vi "Event handler-Z Setup.vi"(8 "error in (no error)":errorcluster, 9 "Obtain Z Stop":bool, 11 "Obtain Z Start":bool) -> (0 "error out":errorcluster)   [LabVIEW 2017]
uses:
  Typedefs/Read Write Enum.ctl
  Global Variables/gl_UI Ctrl Refs.vi
  Global Variables/General Globals.vi
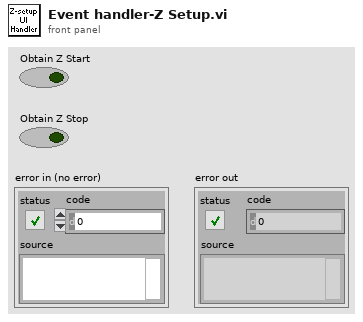
[diagram p1: front panel]
types:
  T1 = typedef "Read Write Enum.ctl" = enum16{"Read", "Write"}
  T2 = typedef "UI ctrl refs cluster.ctl" = cluster{"Top level VI path":path, "Top level VI ref":refnum<vi>, "User menu ref":refnum<k9>, "Sub Panel control":refnum<vi>, "Imaging Param Tab":refnum<vi>, "Occurrence-Start drivers":refnum<k4>, "Occurrence-Speed logging initialised":refnum<k4>, "Occurrence-XYZ stage initialised":refnum<k4>, "Exit button":refnum<vi>, "Status ind":refnum<vi>, "Set as origin":refnum<vi>, "Speed Logging":refnum<vi>, "Time Lapse":refnum<vi>, "Live Imaging":refnum<vi>, "AOL Z Stack":refnum<vi>, "Motor Z Stack":refnum<vi>, "Funct Acq button":refnum<vi>, "Hard Shutter":refnum<vi>, "Virtual Shutter":refnum<vi>, "Laser Power":refnum<vi>, "AOL Mode":refnum<vi>, "Frame Size":refnum<vi>, "Field of View":refnum<vi>, "Dwell Time":refnum<vi>, "Zoom":refnum<vi>, "AOL Z":refnum<vi>, "Objective":refnum<vi>, "Axis":refnum<vi>, "Paths & Names":refnum<vi>, "Experiment folder path (ind.)":refnum<vi>, "Last State (Ind.)":refnum<vi>, "Averages":refnum<vi>, "Angle (degrees)":refnum<vi>, "X centre":refnum<vi>, "Y centre":refnum<vi>, "Plane Mode":refnum<vi>, "# Planes":refnum<vi>, "Z Start":refnum<vi>, "Z Stop":refnum<vi>, "Z Step":refnum<vi>, "PMT 1":refnum<vi>, "PMT 2":refnum<vi>, "Stage XYZ Position":refnum<vi>, "Pockels@Z Start":refnum<vi>, "Pockels@Z Stop":refnum<vi>, "Obtain Z Start":refnum<vi>, "Obtain Z Stop":refnum<vi>, "Live stim.trig.period":refnum<vi>, "Live stim.trig.enable":refnum<vi>, "Movement Correction":refnum<vi>, "Load Reference Image":refnum<vi>, "XY Stage Move":refnum<vi>, "MovCor Cluster":refnum<vi>, "RefDAQParam":refnum<vi>, "Funct. Acq. Pockels Modulation":refnum<vi>, "Ref Laser Power":refnum<vi>, "Enable Video Recording":refnum<vi>, "Video Record-Live Imaging":refnum<vi>, "Video Record-Funct acq":refnum<vi>, "Reference Source":refnum<vi>, "AOL Z-stack Chirps Ready (ind)":refnum<vi>, "Target time between mov.cor. ref triggers (ms)":refnum<vi>, "Funct. Acq. Ref frame save":refnum<vi>, "Tracking button":refnum<vi>, "Show ref plots window":refnum<vi>, "Center freq ind (nm)":refnum<vi>, "Pickup mode (ind)":refnum<vi>, "Logging queue (ind)":refnum<vi>, "Back aperture power (ind.)":refnum<vi>, "Power after objective (ind.)":refnum<vi>, "Switch user":refnum<vi>, "Ls1 Conn. Status":refnum<vi>, "Ls1Tuning Status":refnum<vi>, "Ls1 Faults":refnum<vi>, "Ls1 Connection":refnum<vi>, "Ls1 Mode":refnum<vi>, "Ls1 POWER [mW]":refnum<vi>, "Ls1Shutter":refnum<vi>, "Ls1 Wavelength":refnum<vi>, "Ls1 Note":refnum<vi>, "Ls1 Confirm Wav":refnum<vi>, "Ls1 PreChrp Prism1":refnum<vi>, "Ls1 PreChrp Prism2":refnum<vi>, "Ls1 wav top Ind":refnum<vi>, "Ls1 power top Ind":refnum<vi>, "Ls1 Pump peak Hold":refnum<vi>, "Ls1 Status Ind":refnum<vi>, "Ls1 wav cancel":refnum<vi>, "Experiment Type":refnum<vi>, "Biology Information":refnum<vi>}
  T3 = typedef "Laser control knob.ctl" = u16
  T4 = cluster{"ZStack":cluster{"Zstart":dbl, "Zstop":dbl, "Zstep":dbl}, "Laser Power %":cluster{"@ Start":dbl, "@ Stop":dbl}}
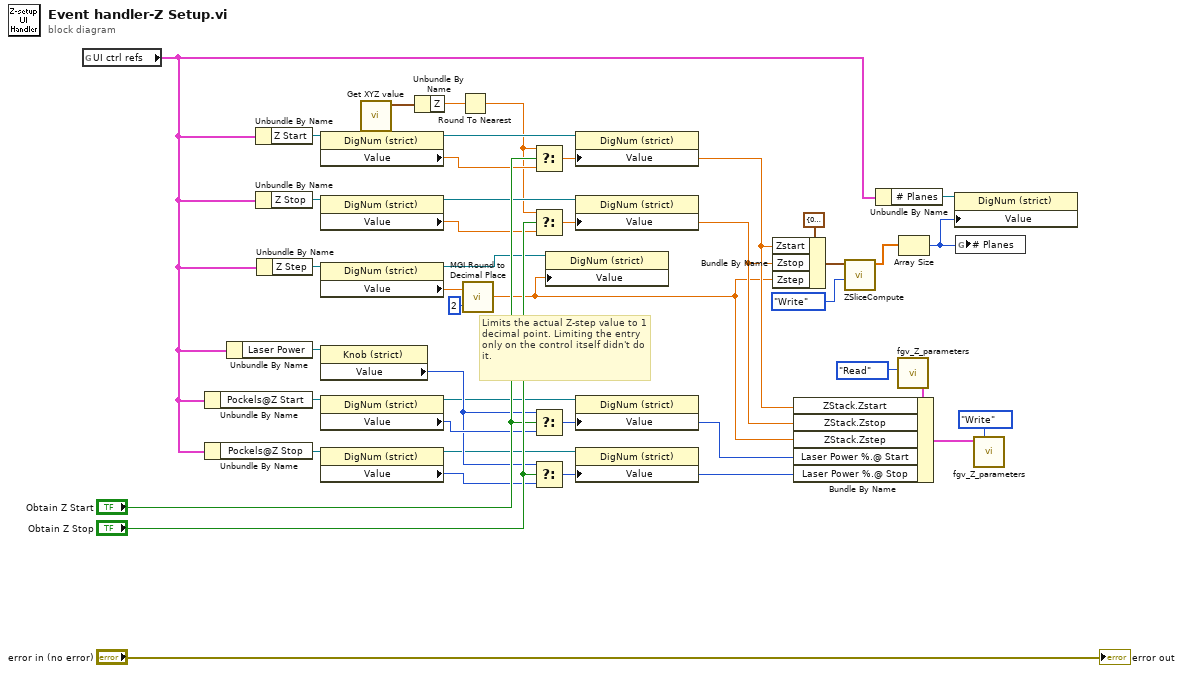
[diagram p0: block diagram]
diagram:
  # "Limits the actual Z-step value to 1 decimal point. Limiting the entry only on the control itself didn't do it."
  n1 = global read "gl_UI Ctrl Refs.vi" "UI ctrl refs"() -> (w38:T2)
  n2 = Unbundle By Name(w38) -> ("Pockels@Z Start"=w16:refnum<vi>)
  n3 = Unbundle By Name(w38) -> ("Pockels@Z Stop"=w15:refnum<vi>)
  n4 = Unbundle By Name(w38) -> ("Laser Power"=w17:refnum<vi>)
  n5 = Unbundle By Name(w38) -> ("Z Start"=w23:refnum<vi>)
  n6 = Unbundle By Name(w38) -> ("Z Stop"=w22:refnum<vi>)
  n7 = Unbundle By Name(w38) -> ("Z Step"=w18:refnum<vi>)
  n8 = property on="Property Node" class="DigNum (strict)"(reference=w23) -> (reference out=w26:refnum<vi>, "Value"=w25:dbl)  [unwired: 1 in, 1 out]
  n9 = property on="Property Node" class="DigNum (strict)"(reference=w22) -> (reference out=w21:refnum<vi>, "Value"=w20:dbl)  [unwired: 1 in, 1 out]
  n10 = property on="Property Node" class="DigNum (strict)"(reference=w18) -> (reference out=w2:refnum<vi>, "Value"=w3:dbl)  [unwired: 1 in, 1 out]
  n11 = property on="Property Node" class="Knob (strict)"(reference=w17) -> ("Value"=w32:T3)  [unwired: 1 in, 2 out]
  n12 = property on="Property Node" class="DigNum (strict)"(reference=w16) -> (reference out=w14:refnum<vi>, "Value"=w33:u16)  [unwired: 1 in, 1 out]
  n13 = property on="Property Node" class="DigNum (strict)"(reference=w15) -> (reference out=w13:refnum<vi>, "Value"=w31:u16)  [unwired: 1 in, 1 out]
  n14 = call "Get XYZ value.vi"() -> ("Stage XYZ Position"=w7:cluster{"X":sgl, "Y":sgl, "Z":sgl})  [unwired: 11 in]
  n15 = Unbundle By Name(w7) -> ("Z"=w34:sgl)
  n16 = Round To Nearest(number=w34) -> (nearest integer value=w5:sgl)
  n17 = call <userlib>:"MGI Round to Decimal Place.vi"("Decimal Digits"=2, "Number"=w3) -> ("Rounded"=w1:dbl)  [unwired: 1 in]
  n18 = Select(t=w5, s="Obtain Z Start", f=w25) -> (s? t:f=w24:dbl)
  n19 = Select(t=w5, s="Obtain Z Stop", f=w20) -> (s? t:f=w19:dbl)
  n20 = Select(t=w32, s="Obtain Z Start", f=w33) -> (s? t:f=w12:T3)
  n21 = Select(t=w32, s="Obtain Z Stop", f=w31) -> (s? t:f=w11:T3)
  n22 = property on="Property Node" class="DigNum (strict)"(reference=w2, "Value"=w1) -> ()  [unwired: 1 in, 2 out]
  n23 = property on="Property Node" class="DigNum (strict)"(reference=w26, "Value"=w24) -> ()  [unwired: 1 in, 2 out]
  n24 = property on="Property Node" class="DigNum (strict)"(reference=w21, "Value"=w19) -> ()  [unwired: 1 in, 2 out]
  n25 = property on="Property Node" class="DigNum (strict)"(reference=w14, "Value"=w12) -> ()  [unwired: 1 in, 2 out]
  n26 = property on="Property Node" class="DigNum (strict)"(reference=w13, "Value"=w11) -> ()  [unwired: 1 in, 2 out]
  n27 = Bundle By Name(cluster=cluster{"Zstart":dbl, "Zstop":dbl, "Zstep":dbl} {"Zstart"=0.0, "Zstop"=0.0, "Zstep"=0.0} ("ZStack"), "Zstart"=w24, "Zstop"=w19, "Zstep"=w1) -> (w36:cluster{"Zstart":dbl, "Zstop":dbl, "Zstep":dbl})
  n28 = call "ZSliceCompute.vi"("Function"=Read_Write_Enum."Write", "ZStack (um)"=w36) -> ("Motor Z Planes(um)"=w35:dbl[])  [unwired: 6 in, 3 out]
  n29 = Unbundle By Name(w38) -> ("# Planes"=w10:refnum<vi>)
  n30 = call "fgv_Z_parameters.vi"("Function"=enum16{"Intialize", "Write", "Read", "Clear"}."Read") -> ("Z Parameters"=w28:T4)  [unwired: 9 in, 1 out]
  n31 = Bundle By Name(cluster=w28, "ZStack.Zstart"=w24, "ZStack.Zstop"=w19, "ZStack.Zstep"=w1, "Laser Power %.@ Start"=w12, "Laser Power %.@ Stop"=w11) -> (w27:T4)
  n32 = Array Size(array=w35) -> (size(s)=w8:i32)
  n33 = property on="Property Node" class="DigNum (strict)"(reference=w10, "Value"=w8) -> ()  [unwired: 1 in, 2 out]
  n34 = global write "General Globals.vi" "# Planes"(w8) -> ()
  n35 = call "fgv_Z_parameters.vi"("Function"=enum16{"Intialize", "Write", "Read", "Clear"}."Write", "Z Parameters"=w27) -> ()  [unwired: 8 in, 2 out]
  "error out" <- "error in (no error)"
